vi "Define Display Columns.vi"(11 "Enum in":refnum<vi>) -> (3 "Columns":T1[](array[typedef]) {"MinWidth" min=2 step=1; "AutoSizeMode" items=["None"=1, "ColumnHeader"=2, "AllCellsExceptHeader"=4, "AllCells"=6, "DisplayedCellsExceptHeader"=8, "DisplayedCells"=10, "Fill"=16]; "FillWeight" min=1 max=100})   [LabVIEW 2013, in "Scaling editor node.lvclass"]
uses:
  Scaling editor node.lvclass
  <vilib>/NI/DCAF Table API/Column/Column Descriptor.ctl
  <vilib>/NI/DCAF Table API/Column/Column Type.ctl
  <vilib>/NI/Tag Bus/tag/Data Type.ctl
  <vilib>/NI/DCAF Table API/Table Manager/Call Back Ref Type Def.ctl
  <vilib>/NI/Tag Bus Data Framework/Configuration Editor/Classes/Engine Parent/Engine Parent Editor Node.lvclass
  table callbacks/Change Input DT.vi
  table callbacks/Change Input Tag.vi
  table callbacks/Change Output DT.vi
  table callbacks/Change Output Tag.vi
  <vilib>/NI/Tag Bus Data Framework/Configuration Editor/Classes/Module editor node/module editor node.lvclass
  <vilib>/NI/DCAF Table API/Mapping Column/Mapping Column.lvclass
  <vilib>/NI/Tag Bus/tag/tag descriptor.lvclass
  <vilib>/NI/DCAF Table API/Table Manager/Table Manager.lvclass
  <vilib>/NI/DCAF Table API/Column/Column.lvclass
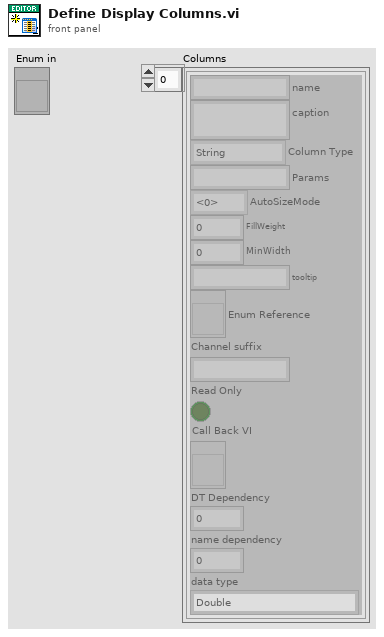
[diagram p1: front panel]
types:
  T1 = typedef "Table Manager.lvlib/Column.lvclass/Column Descriptor.ctl" = cluster{"name":string, "caption":string, "Column Type":T2, "Params":string, "AutoSizeMode":i32, "FillWeight":sgl, "MinWidth":u32, "tooltip":string, "Enum Reference":refnum<vi>, "Channel suffix":string, "Read Only":bool, "Call Back VI":T3, "DT Dependency":i32, "name dependency":i32, "data type":T4}
  T2 = typedef "Table Manager.lvlib/Column.lvclass/Column Type.ctl" = enum16{"String", "Mapping", "Channel Name", "Tag", "Enum", "Data Type", "Numeric"}
  T3 = typedef "Table Manager.lvlib/Table Manager.lvclass/Call Back Ref Type Def.ctl" = refnum<vi>
  T4 = typedef "tag bus.lvlib/tag descriptor.lvclass/Data Type.ctl" = enum16{"Double", "Single", "I64", "I32", "I16", "I8", "U64", "U32", "U16", "U8", "Boolean", "String", "Array of Double", "Array of Single", "Array of I64", "Array of I32", "Array of I16", "Array of I8", "Array of U64", "Array of U32", "Array of U16", "Array of U8", "Array of Boolean", "Array of String"}
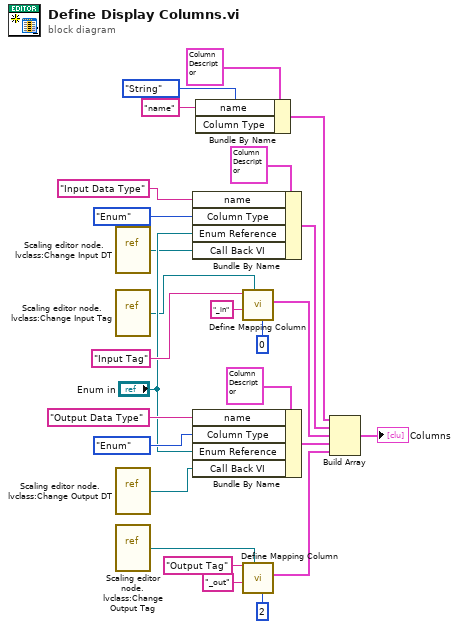
[diagram p0: block diagram]
diagram:
  n1 = vi-ref "Scaling editor node.lvclass:Change Input DT.vi"() -> (w10:refnum<vi>)
  n2 = vi-ref "Scaling editor node.lvclass:Change Input Tag.vi"() -> (w9:refnum<vi>)
  n3 = vi-ref "Scaling editor node.lvclass:Change Output DT.vi"() -> (w7:refnum<vi>)
  n4 = vi-ref "Scaling editor node.lvclass:Change Output Tag.vi"() -> (w8:refnum<vi>)
  n5 = Bundle By Name(cluster=T1 {"name"="Link", "caption"="", "Column Type"=enum."String", "Params"="", "AutoSizeMode"=1, "FillWeight"=100.0, "MinWidth"=50, "tooltip"="The quick brown fox jumps over the lazy dog", "Enum Reference"=refnum, "Channel suffix"="", "Read Only"=FALSE, "Call Back VI"=refnum, "DT Dependency"=0, "name dependency"=0, "data type"=enum."Double"} ("Table Manager.lvlib:Column.lvclass:Column Descriptor"), "name"="Input Data Type", "Column Type"=Column_Type."Enum", "Enum Reference"="Enum in", "Call Back VI"=w10) -> (w14:T1)
  n6 = Bundle By Name(cluster=T1 {"name"="Link", "caption"="", "Column Type"=enum."String", "Params"="", "AutoSizeMode"=1, "FillWeight"=100.0, "MinWidth"=50, "tooltip"="The quick brown fox jumps over the lazy dog", "Enum Reference"=refnum, "Channel suffix"="", "Read Only"=FALSE, "Call Back VI"=refnum, "DT Dependency"=0, "name dependency"=0, "data type"=enum."Double"} ("Table Manager.lvlib:Column.lvclass:Column Descriptor"), "name"="Output Data Type", "Column Type"=Column_Type."Enum", "Enum Reference"="Enum in", "Call Back VI"=w7) -> (w12:T1)
  n7 = Bundle By Name(cluster=T1 {"name"="Link", "caption"="", "Column Type"=enum."String", "Params"="", "AutoSizeMode"=1, "FillWeight"=100.0, "MinWidth"=50, "tooltip"="The quick brown fox jumps over the lazy dog", "Enum Reference"=refnum, "Channel suffix"="", "Read Only"=FALSE, "Call Back VI"=refnum, "DT Dependency"=0, "name dependency"=0, "data type"=enum."Double"} ("Table Manager.lvlib:Column.lvclass:Column Descriptor"), "name"="name", "Column Type"=Column_Type."String") -> (w3:T1)
  n8 = call <vilib>:"Define Mapping Column.vi"("DT Dependency"=0, "Call Back VI"=w9, "Channel suffix"="_in", "name"="Input Tag") -> ("Table Manager.lvlib:Column.lvclass:Column Descriptor"=w13:T1)  [unwired: 7 in]
  n9 = call <vilib>:"Define Mapping Column.vi"("DT Dependency"=2, "Call Back VI"=w8, "Channel suffix"="_out", "name"="Output Tag") -> ("Table Manager.lvlib:Column.lvclass:Column Descriptor"=w11:T1)  [unwired: 7 in]
  n10 = Build Array(w3, w14, w13, w12, w11) -> (→"Columns":T1[])
